vi "Spectrum Processing.vi"(0 "VISA resource name":refnum<visa-resource-name>, 1 "Spectral Mode (0:Absorbance)":u16(ring) items=["Absorbance", "Transmission", "Irradiance"], 5 "Sample Spectrum":dbl[](array[numeric]), 7 "Reference Spectrum":dbl[](array[numeric]), 9 "Dark Spectrum":dbl[](array[numeric]), 11 "error in (no error)":errorcluster, 12 "Wavelength (nm)":dbl[](array[numeric]), 13 "Color Temperature (2850 K)":dbl=2850.0) -> (4 "VISA resource name out":refnum<visa-resource-name>, 8 "Processed Spectrum":dbl[](array[numeric]), 15 "error out":errorcluster)   [LabVIEW 2013, in "Ocean Optics 2000 4000.lvlib"]
doc: "Converts normal spectrum to absorbance, transmission or relative irradiance. A sample, reference and dark spectrum is needed for these calculations.\n\n<b>Absorbance</b> - generally used to measure, on a logarithmic scale, how much light from a source was absorbed by a surface, liquid, or gas. \n<b>Transmission</b> - a simple measurement that calculates how much light from the light source was transmitted through a particular material (solid, liquid, or gas) usually as a percentage\n<b>Relative Irradiance</b> - Relative irradiance corrects the shape of a measured spectrum to account for inefficiencies in the optics and detector of a spectrometer. The shape is altered to match that of an ideal \"blackbody\" emission source; basically, any thing that is heated enough will start to emit energy, some of which may be visible light. Using a light source that is close to an ideal blackbody in its actual emission, the spectrum shape is corrected to match the shape of a theoretical blackbody at the same temperature."
uses:
  <instrlib>/Ocean Optics 2000 4000/Ocean Optics 2000 4000.lvlib
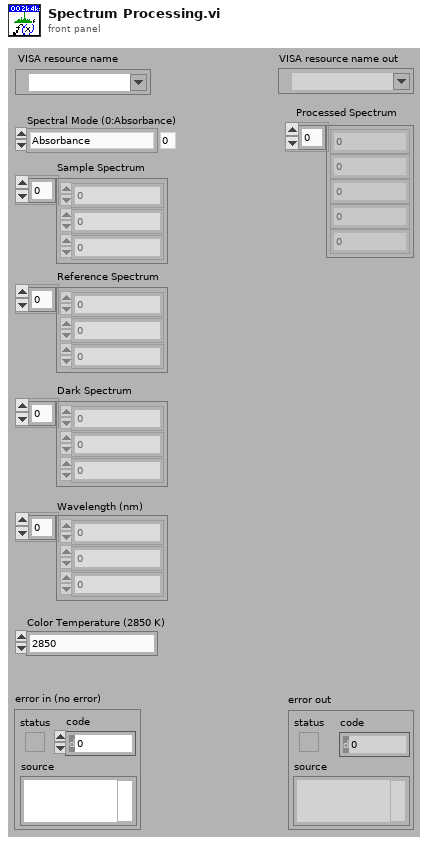
[diagram p1: front panel]
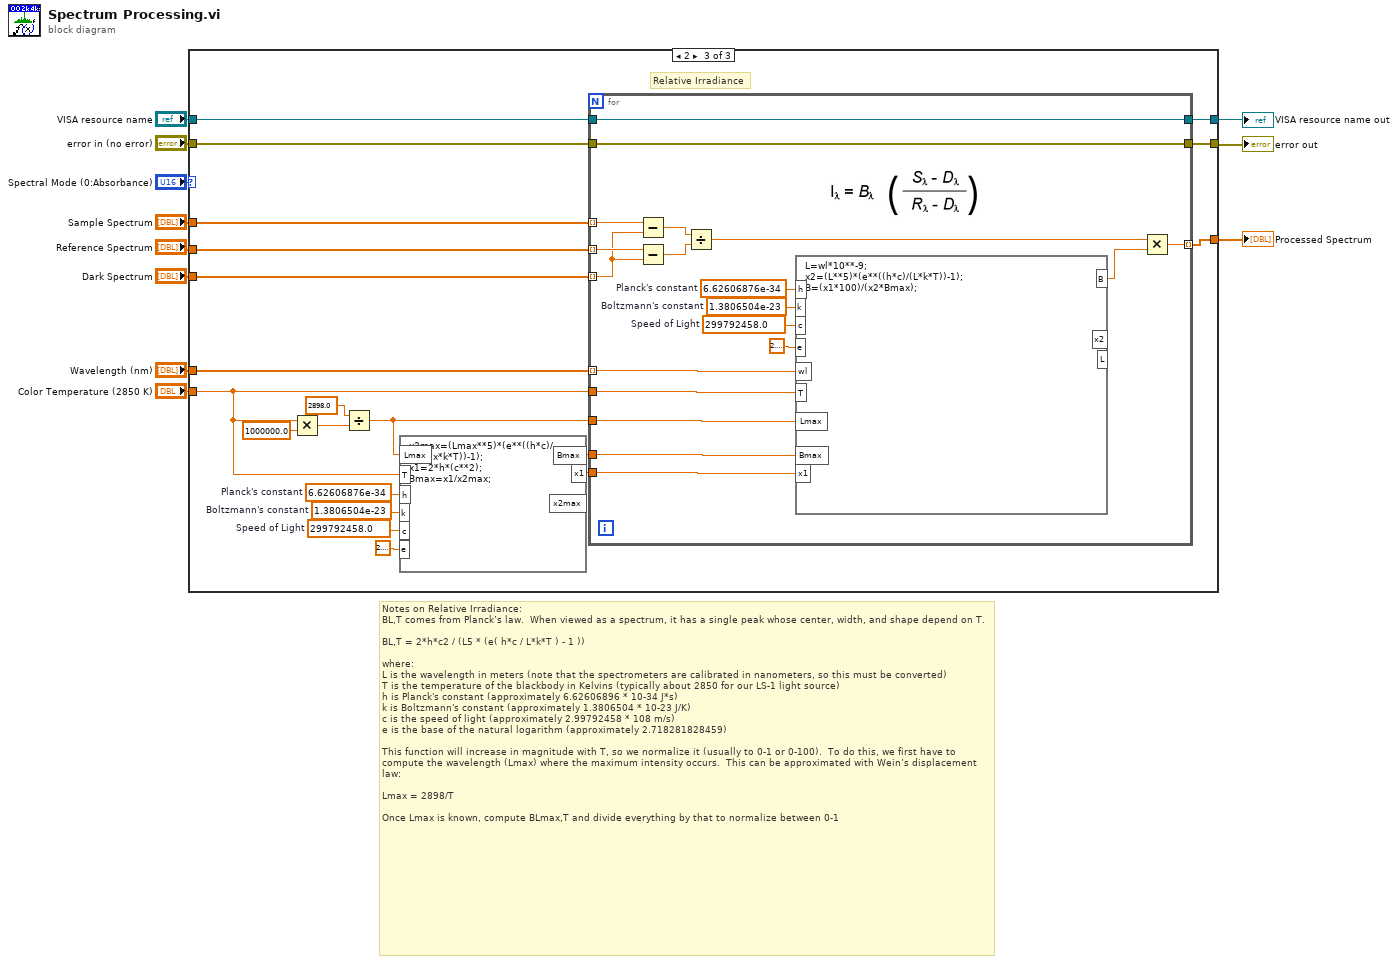
[diagram p0: block diagram]
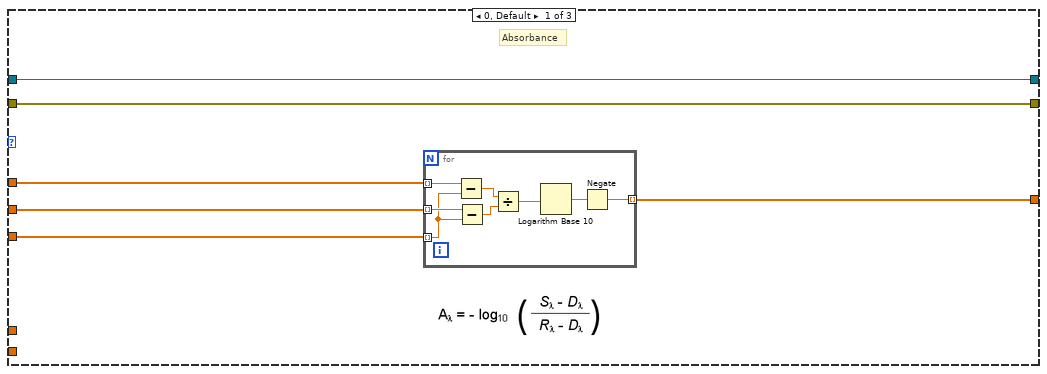
[diagram p2: hidden frame]
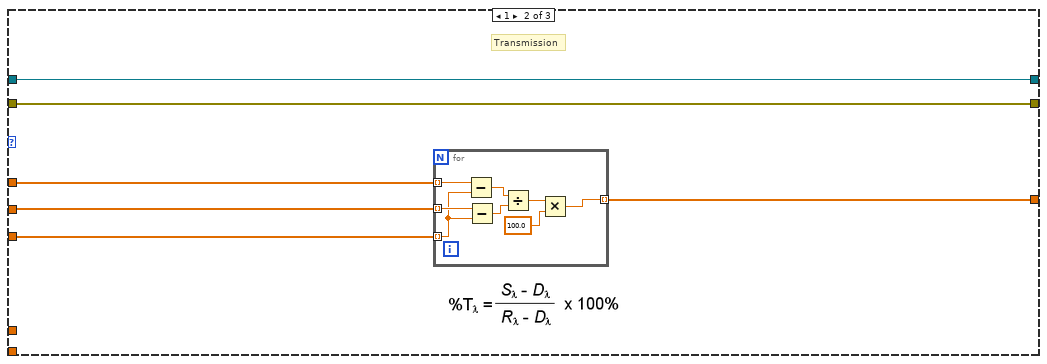
[diagram p3: hidden frame]
diagram:
  # "Notes on Relative Irradiance: \nBL,T comes from Planck’s law.  When viewed as a spectrum, it has a single peak whose center, width, and shape depend on T. \n\nBL,T = 2*h*c2 / (L5 * (e( h*c / L*k*T ) - 1 ))\n\nwhere:\nL is the wavelength in meters (note that the spectrometers are calibrated in nanometers, so this must be converted)\nT is the temperature of the blackbody in Kelvins (typically about 2850 for our LS-1 light source)\nh is Planck's constant (approximately 6.62606896 * 10-34 J*s)\nk is Boltzmann's constant (approximately 1.3806504 * 10-23 J/K)\nc is the speed of light (approximately 2.99792458 * 108 m/s)\ne is the base of the natural logarithm (approximately 2.718281828459) \n  \nThis function will increase in magnitude with T, so we normalize it (usually to 0-1 or 0-100).  To do this, we first have to compute the wavelength (Lmax) where the maximum intensity occurs.  This can be approximated with Wein’s displacement law: \n  \nLmax = 2898/T  \n  \nOnce Lmax is known, compute BLmax,T and divide everything by that to normalize between 0-1"
  n1 = case shown="2" "Spectral Mode (0:Absorbance)" {
    tunnel: "Sample Spectrum" -> [w17 w31 w53]
    tunnel: "Reference Spectrum" -> [w15 w30 w51]
    tunnel: "Dark Spectrum" -> [w16 w29 w52]
    tunnel: [w12 w28 w58] -> w6
    tunnel: "VISA resource name" -> [w14 w27 w57]
    tunnel: "error in (no error)" -> [w13 w26 w54]
    tunnel: [w14 w27 w56] -> w8
    tunnel: [w13 w26 w55] -> w7
    tunnel: "Wavelength (nm)" -> [_ _ w59]
    tunnel: "Color Temperature (2850 K)" -> [_ _ w42]
    frame 0, Default {
      # "Absorbance"
      n2 = for {
        tunnel: w17 -> [w25] mode=indexing
        tunnel: w15 -> [w24] mode=indexing
        tunnel: w16 -> [w23] mode=indexing
        tunnel: [w18] -> w12 mode=indexing
        n3 = Subtract(x=w25, y=w23) -> (x-y=w21:dbl)
        n4 = Subtract(x=w24, y=w23) -> (x-y=w20:dbl)
        n5 = Divide(x=w21, y=w20) -> (x/y=w22:dbl)
        n6 = Logarithm Base 10(1:w22) -> (0:w19:dbl)
        n7 = Negate(x=w19) -> (-x=w18:dbl)
      }
    }
    frame 1 {
      # "Transmission"
      n8 = for {
        tunnel: w31 -> [w39] mode=indexing
        tunnel: w30 -> [w38] mode=indexing
        tunnel: w29 -> [w37] mode=indexing
        tunnel: [w32] -> w28 mode=indexing
        n9 = Subtract(x=w39, y=w37) -> (x-y=w36:dbl)
        n10 = Subtract(x=w38, y=w37) -> (x-y=w35:dbl)
        n11 = Divide(x=w36, y=w35) -> (x/y=w34:dbl)
        n12 = Multiply(x=w34, y=100.0) -> (x*y=w32:dbl)
      }
    }
    frame 2 {
      w46 = 299792458.0  # Speed of Light
      w45 = 1.3806504e-23  # Boltzmann's constant
      w44 = 6.62606876e-34  # Planck's constant
      # "Relative Irradiance"
      n13 = Multiply(x=w42, y=1000000.0) -> (x*y=w49:dbl)
      n14 = Divide(x=2898.0, y=w49) -> (x/y=w43:dbl)
      n15 = formula code="x2max=(Lmax**5)*(e**((h*c)/(Lmax*k*T))-1);\nx1=2*h*(c**2);\nBmax=x1/x2max;"("h"=w44, "k"=w45, "c"=w46, "Lmax"=w43, "e"=2.718281828459045, "T"=w42) -> ("x1"=w40:dbl, "Bmax"=w41:dbl)  [unwired: 1 out]
      n16 = for {
        tunnel: w59 -> [w78] mode=indexing
        tunnel: w42 -> [w77]
        tunnel: [w64] -> w58 mode=indexing
        tunnel: [w72] -> w56
        tunnel: w57 -> [w72]
        tunnel: [w71] -> w55
        tunnel: w54 -> [w71]
        tunnel: w53 -> [w70] mode=indexing
        tunnel: w52 -> [w68] mode=indexing
        tunnel: w51 -> [w69] mode=indexing
        tunnel: w43 -> [w62]
        tunnel: w41 -> [w60]
        tunnel: w40 -> [w61]
        w74 = 299792458.0  # Speed of Light
        w75 = 1.3806504e-23  # Boltzmann's constant
        w76 = 6.62606876e-34  # Planck's constant
        n17 = Subtract(x=w70, y=w68) -> (x-y=w67:dbl)
        n18 = Subtract(x=w69, y=w68) -> (x-y=w66:dbl)
        n19 = Divide(x=w67, y=w66) -> (x/y=w63:dbl)
        n20 = formula code="L=wl*10**-9;\nx2=(L**5)*(e**((h*c)/(L*k*T))-1);\nB=(x1*100)/(x2*Bmax);"("wl"=w78, "T"=w77, "x1"=w61, "h"=w76, "k"=w75, "c"=w74, "e"=2.718281828459045, "Lmax"=w62, "Bmax"=w60) -> ("B"=w65:dbl)  [unwired: 2 out]
        n21 = Multiply(x=w63, y=w65) -> (x*y=w64:dbl)
      }
    }
  }
  "VISA resource name out" <- w8
  "error out" <- w7
  "Processed Spectrum" <- w6
